vi "unlock.vi"(8 "error in":errorcluster, 11 "connection ID":refnum<k5>) -> (0 "error out":errorcluster, 3 "connection ID":refnum<k5>)   [LabVIEW 2015]
panel:
  in  "Set Command":string="unlock"
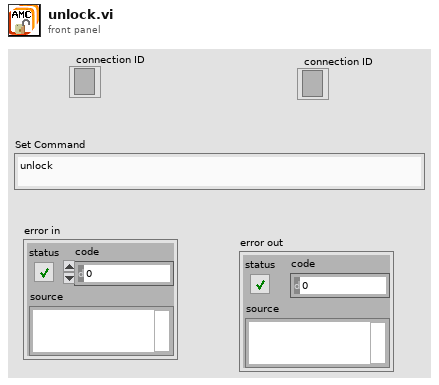
[diagram p1: front panel]
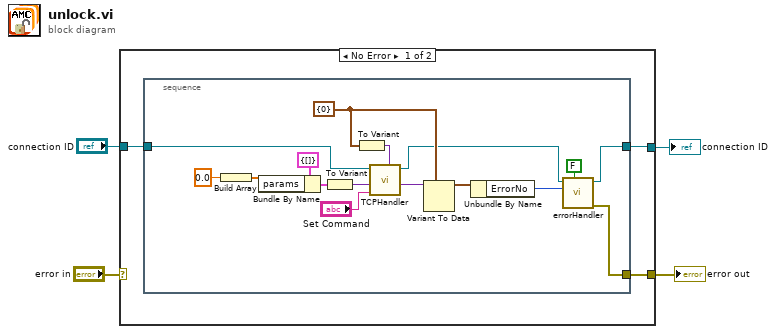
[diagram p0: block diagram]
diagram:
  n1 = case shown="No Error" "error in" {
    selector: "error in" -> [_ w24]
    tunnel: [w5 w24] -> w4
    tunnel: [w6 w25] -> w3
    tunnel: "connection ID" -> [w7 w25]
    frame No Error {
      n2 = stacked-sequence {
        tunnel: [w8] -> w6
        tunnel: w7 -> [w14]
        tunnel: [w15] -> w5
        frame #0 {
          w12 = cluster{"ErrorNo":i32} {"ErrorNo"=0} ("input cluster")
          n3 = Build Array(0.0 ("element")) -> (w19:dbl[])
          n4 = Bundle By Name(cluster=cluster{"params":i32[]} {"params"=[]} ("input cluster"), "params"=w19) -> (w20:cluster{"params":i32[]})
          n5 = To Variant(anything=w20) -> (Variant=w21:variant)
          n6 = To Variant(anything=w12) -> (Variant=w13:variant)
          n7 = call "TCPHandler.vi"("result Types"=w13, "method"="Set Command", "params"=w21, "connection ID"=w14) -> ("result"=w17:variant, "connection ID"=w9:refnum<k5>)  [unwired: 5 in, 1 out]
          n8 = Variant To Data(type=w12, Variant=w17) -> (data=w22:cluster{"ErrorNo":i32})  [unwired: 1 in, 1 out]
          n9 = Unbundle By Name(w22) -> ("ErrorNo"=w23:i32)
          n10 = call "errorHandler.vi"("show popup"=FALSE, "error number"=w23, "connection ID"=w9) -> ("error out"=w15:errorcluster, "connection ID"=w8:refnum<k5>)  [unwired: 7 in]
        }
      }
    }
    frame Error {
    }
  }
  "error out" <- w4
  "connection ID" <- w3
